vi "Lockin - Format Results.vi"(8 "error in (no error)":errorcluster, 10 "signal in":waveform(dbl)[](array[waveform]), 11 "Lockin.DAQ":refnum<class "Lockin.DAQ.lvclass">) -> (0 "error out":errorcluster, 1 "SweepResults":T1, 2 "Results (X,Y,R,Theta)":dbl[][](array[numeric]), 3 "Lockin.DAQ":refnum<class "Lockin.DAQ.lvclass">)   [LabVIEW 2019, in "Lockin.DAQ.lvclass"]
uses:
  Lockin.DAQ.lvclass
  Typedefs/SweepResults--Cluster.ctl
  <vilib>/measure/maresamp.llb/Resample Waveform (single shot).vi
  <vilib>/measure/NI_MAPro.lvlib
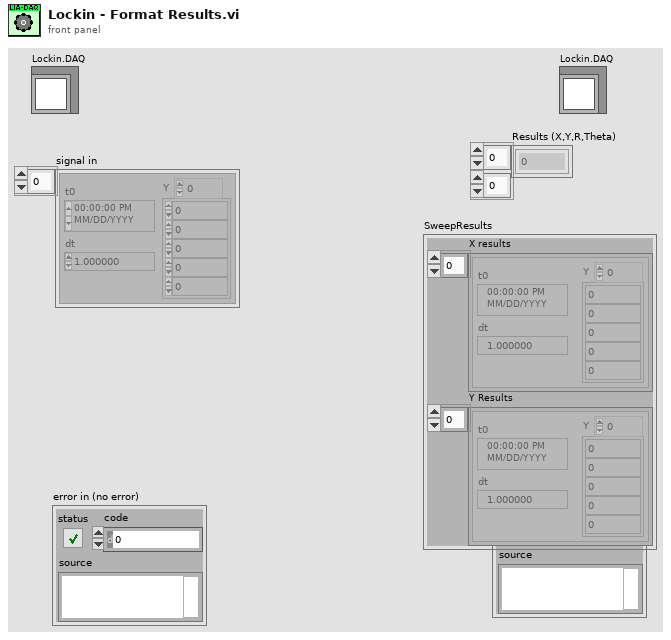
[diagram p1: front panel]
types:
  T1 = typedef "Lockin.DAQ.lvclass/SweepResults--Cluster.ctl" = cluster{"X results":waveform(dbl)[], "Y Results":waveform(dbl)[]}
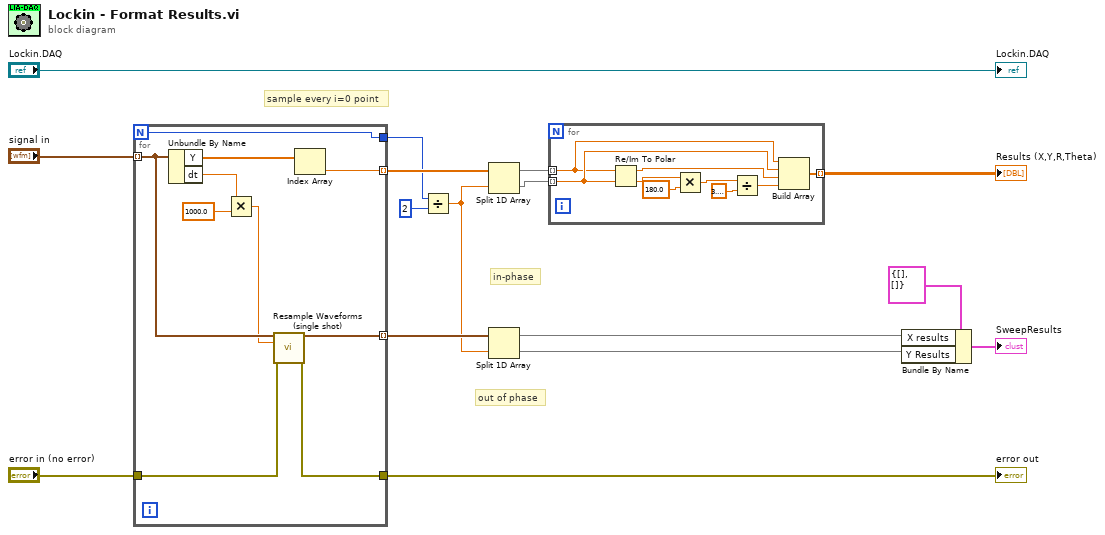
[diagram p0: block diagram]
diagram:
  # "in-phase"
  # "out of phase"
  # "sample every i=0 point"
  n1 = for {
    N -> [w24]
    tunnel: "signal in" -> [w21] mode=indexing
    tunnel: [w26] -> w14 mode=indexing
    tunnel: [w24] -> w13
    tunnel: [w23] -> w11 mode=indexing
    tunnel: "error in (no error)" -> [w18]
    tunnel: [w17] -> w5
    n2 = Unbundle By Name(w21) -> ("Y"=w25:dbl[], "dt"=w20:dbl)
    n3 = Multiply(x=w20, y=1000.0) -> (x*y=w19:dbl)
    n4 = call-poly <vilib>:"Resample Waveforms (single shot).vi"("waveform in"=w21, "dt"=w19, "error in (no error)"=w18) -> ("resampled waveform out"=w23:waveform(dbl), "error out"=w17:errorcluster)  [unwired: 9 in, 2 out]
    n5 = Index Array(array=w25) -> (element=w26:dbl)  [unwired: 1 in]
  }
  "error out" <- w5
  n6 = Divide(x=w13, y=2) -> (x/y=w10:dbl)
  n7 = Split 1D Array(array=w14, index=w10) -> (first subarray=w4:dbl[], second subarray=w3:dbl[])
  n8 = Split 1D Array(array=w11, index=w10) -> (first subarray=w2:waveform(dbl)[], second subarray=w1:waveform(dbl)[])
  n9 = for {
    tunnel: w4 -> [w27] mode=indexing
    tunnel: w3 -> [w29] mode=indexing
    tunnel: [w35] -> w16 mode=indexing
    n10 = Re/Im To Polar(2:w29, 3:w27) -> (0:w33:dbl, 1:w28:dbl)
    n11 = Multiply(x=w33, y=180.0) -> (x*y=w34:dbl)
    n12 = Divide(x=w34, y=3.141592653589793) -> (x/y=w30:dbl)
    n13 = Build Array(w27, w29, w28, w30) -> (w35:dbl[])
  }
  "Results (X,Y,R,Theta)" <- w16
  n14 = Bundle By Name(cluster=T1 {"X results"=[], "Y Results"=[]} ("SweepResults"), "X results"=w2, "Y Results"=w1) -> (→"SweepResults":T1)
  "Lockin.DAQ" <- "Lockin.DAQ"
